vi "GET_Glyphs [].vi"(8 "error in (no error)":errorcluster, 11 "Glyph.lvclass in":refnum<class "Glyph.lvclass">) -> (0 "error out":errorcluster, 2 "Glyphs []":T1[](array[typedef]), 3 "Glyph.lvclass out":refnum<class "Glyph.lvclass">)   [LabVIEW 2020, in "Glyph.lvclass"]
uses:
  Glyph.lvclass
  Glyph.lvclass/Glyph.ctl
  vi.lib/LabVIEW Icon API/lv_icon/Controls/Graphic.ctl
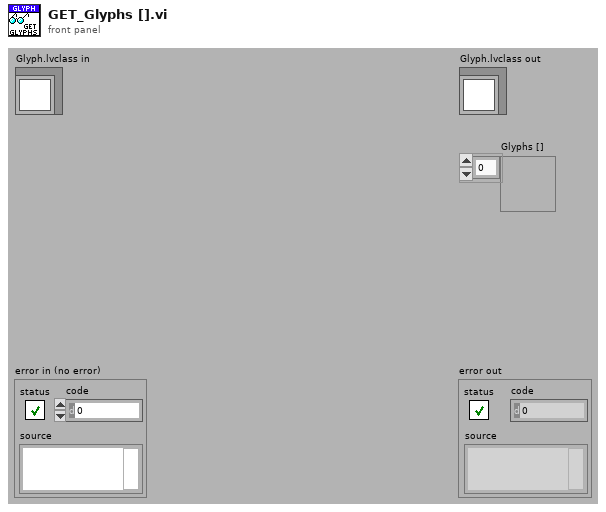
[diagram p1: front panel]
types:
  T1 = typedef "Graphic.ctl" = cluster{"Rectangle":cluster{"left":i16, "top":i16, "right":i16, "bottom":i16}, "Path":path, "Image":picture, "Filter":string, "FileName":string}
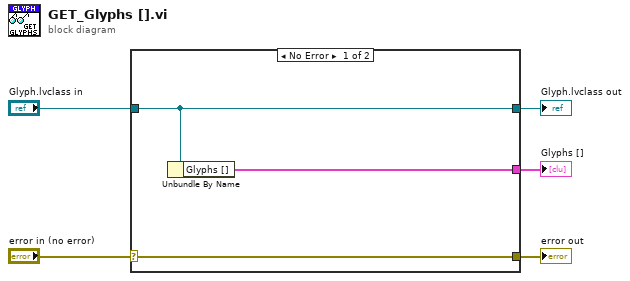
[diagram p0: block diagram]
diagram:
  n1 = case shown="No Error" "error in (no error)" {
    selector: "error in (no error)" -> [w8 w9]
    tunnel: [w8 w9] -> w4
    tunnel: [w7 w10] -> w2
    tunnel: "Glyph.lvclass in" -> [w7 w10]
    tunnel: [w6 _] -> w1
    frame No Error {
      n2 = Unbundle By Name(w7) -> ("Glyphs []"=w6:T1[])
    }
    frame Error {
    }
  }
  "error out" <- w4
  "Glyph.lvclass out" <- w2
  "Glyphs []" <- w1
